vi "Assert Channels Are Unique.vi"(8 "error in (no error)":errorcluster, 10 "Channels in":string[](array[string]), 11 "System Monitor System Tests in":refnum<class "System Monitor System Tests.lvclass">) -> (0 "error out":errorcluster, 3 "System Monitor System Tests out":refnum<class "System Monitor System Tests.lvclass">)   [LabVIEW 2027, in "System Monitor System Tests.lvclass"]
uses:
  System Monitor System Tests.lvclass
  <vilib>/NI VeriStand/Execution/Workspace/NI VeriStand - Get Multiple Channel Values.vi
  <vilib>/NI VeriStand/Execution/Workspace/NI_VS Workspace ExecutionAPI.lvlib
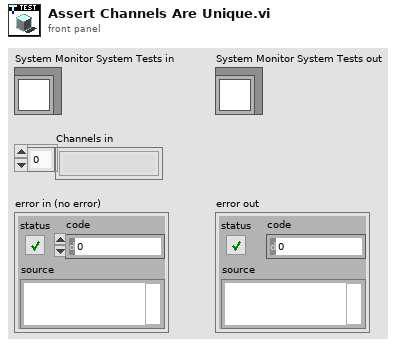
[diagram p1: front panel]
types:
  T1 = typedef "NI_VS Workspace ExecutionAPI.lvlib/WorkspaceAPI.ctl" = refnum<k39>
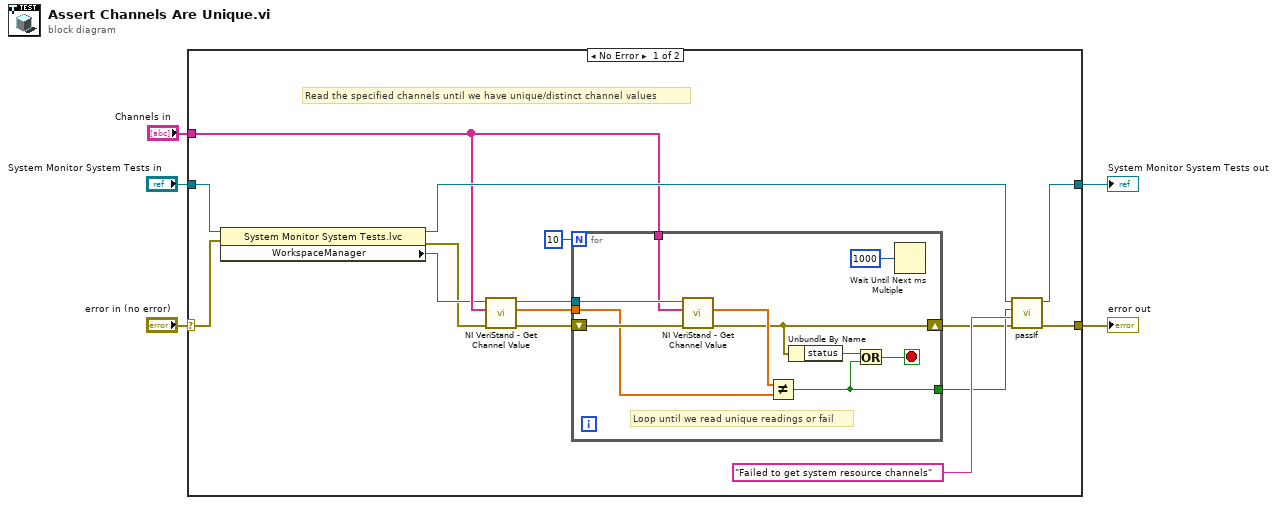
[diagram p0: block diagram]
diagram:
  n1 = case shown="No Error" "error in (no error)" {
    selector: "error in (no error)" -> [w6 w31]
    tunnel: [w18 w32] -> w5
    tunnel: [w16 w31] -> w4
    tunnel: "Channels in" -> [w13 _]
    tunnel: "System Monitor System Tests in" -> [w7 w32]
    frame No Error {
      # "Read the specified channels until we have unique/distinct channel values"
      n2 = property class="System Monitor System Tests.lvc"(reference=w7, error in=w6) -> (reference out=w17:refnum<class "System Monitor System Tests.lvclass">, error out=w8:errorcluster, "WorkspaceManager"=w11:T1)
      n3 = call-poly <vilib>:"NI VeriStand - Get Channel Value.vi"("error in (no error)"=w8, "Channels"=w13, "WorkspaceManager in"=w11) -> ("error out"=w10:errorcluster, "Values"=w14:dbl[], "WorkspaceManager out"=w12:T1)  [unwired: 6 in]
      n4 = for {
        N: 10 -> [_]
        tunnel: w12 -> [w30]
        shift-right: [w24] -> w15
        shift-left: w10 -> [w29]
        tunnel: w13 -> [w28]
        tunnel: w14 -> [w25]
        tunnel: [w22] -> w19
        stop <- w21 stop-if-true
        # "Loop until we read unique readings or fail"
        n5 = call-poly <vilib>:"NI VeriStand - Get Channel Value.vi"("error in (no error)"=w29, "Channels"=w28, "WorkspaceManager in"=w30) -> ("error out"=w24:errorcluster, "Values"=w26:dbl[])  [unwired: 6 in, 1 out]
        n6 = Not Equal?(x=w26, y=w25) -> (x != y?=w22:bool)
        n7 = Unbundle By Name(w24) -> ("status"=w23:bool)
        n8 = Or(x=w23, y=w22) -> (x .or. y?=w21:bool)
        n9 = Wait Until Next ms Multiple(millisecond multiple=u32 1000 ("milliseconds to wait")) -> ()  [unwired: 1 out]
      }
      n10 = call-dynamic "passIf.vi"("error in (no error)"=w15, "message (\"\")"="Failed to get system resource channels" ("message (\"\")"), "pass"=w19, "TestCase in"=w17) -> ("error out"=w16:errorcluster, "TestCase out"=w18:refnum<class "System Monitor System Tests.lvclass">)  [unwired: 6 in]
    }
    frame Error {
    }
  }
  "System Monitor System Tests out" <- w5
  "error out" <- w4
